vi "Destroy.vi"(11 "jettl in":refnum<class "jettl.lvclass">) -> (3 "jettl out":refnum<class "jettl.lvclass">)   [LabVIEW 2021, in "jettl.lvlib" / "jettl.lvclass"]
uses:
  jettl.lvclass
  C:/git/jettl/src/jettl/Actor/Actor.lvclass
  State/Destroy State/Destroy State.lvclass
  C:/git/jettl/src/jettl/jettl/State/State/State.lvclass
  jettl.lvclass/jettl.ctl
  State/State/State.lvclass
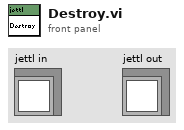
[diagram p1: front panel]
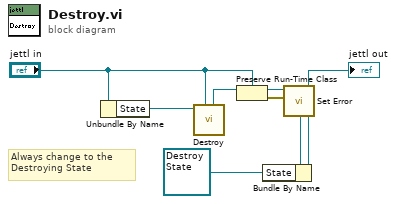
[diagram p0: block diagram]
diagram:
  # "Always change to the Destroying State"
  n1 = Unbundle By Name("jettl in") -> ("State"=w7:refnum<class "State.lvclass">)
  n2 = call-dynamic "Destroy.vi"("Actor in"="jettl in", "State in"=w7) -> ("Actor out"=w5:refnum<class "Actor.lvclass">)  [unwired: 9 in]
  n3 = Preserve Run-Time Class(object in=w5, 2:"jettl in") -> (object out=w3:refnum<class "jettl.lvclass">, error out=w1:errorcluster)  [unwired: 1 in]
  n4 = call-dynamic "Set Error.vi"("Error"=w1, "jettl in"=w3) -> ("jettl out"=w2:refnum<class "jettl.lvclass">)  [unwired: 9 in]
  n5 = Bundle By Name(cluster=w2, "State"=refnum<class "Destroy State.lvclass"> refnum ("LVCAM.lvlib:Destroying Self Actor State.lvclass")) -> (→"jettl out":refnum<class "jettl.lvclass">)
